vi "Main.vi"(11 "Error In":errorcluster) -> (15 "Error Out":errorcluster)   [LabVIEW 2022 SP3]
doc: "This VI has subpanel for sender and receiver. User can select the data type and transmission type for which communication has to take place from sender to receiver."
uses:
  Controls/Operation.ctl
  Controls/State Cluster.ctl
  Controls/Main Data Cluster.ctl
  Classes/Sender/Sender UI.vi
  Classes/Sender/Sender.lvclass
  Classes/Receiver/Receiver UI.vi
  Classes/Receiver/Receiver.lvclass
  Controls/User Event Operation.ctl
  Downloads/Sample PC Template/Sample PC Template/Typedefs/Data.ctl
  Downloads/Sample PC Template/Sample PC Template/Sample PC Template.lvlib
panel:
  in  "Help Button":bool
  # "Sender to Receiver Data Communication Model"
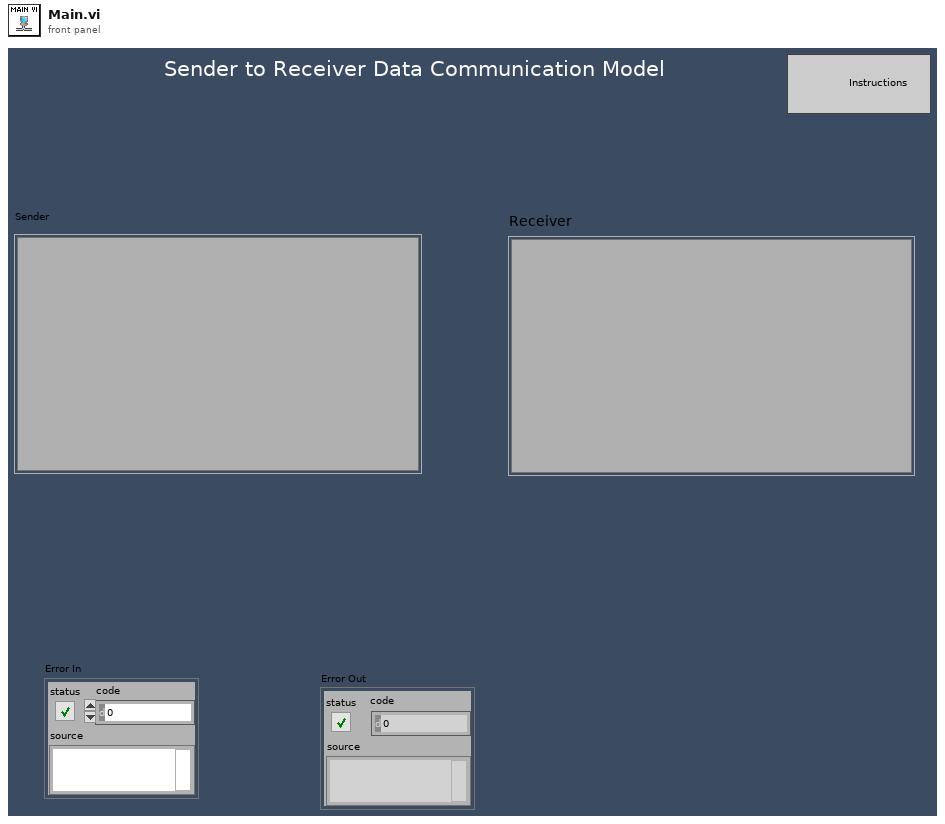
[diagram p1: front panel]
types:
  T1 = typedef "State Cluster.ctl" = cluster{"State":string, "Data":variant}
  T2 = typedef "Operation.ctl" = enum16{"Create", "Enqueue", "Enqueue N", "Enstack", "Dequeue", "Flush", "Release"}
  T3 = typedef "Sample PC Template.lvlib/Data.ctl" = cluster{"State":string, "Data":variant}
  T4 = typedef "User Event Operation.ctl" = enum16{"Obtain", "Generate", "Release"}
  T5 = typedef "Main Data Cluster.ctl" = cluster{"user event out":refnum<user-event>, "Sender Refnum":refnum<vi>, "Receiver refnum":refnum<vi>}
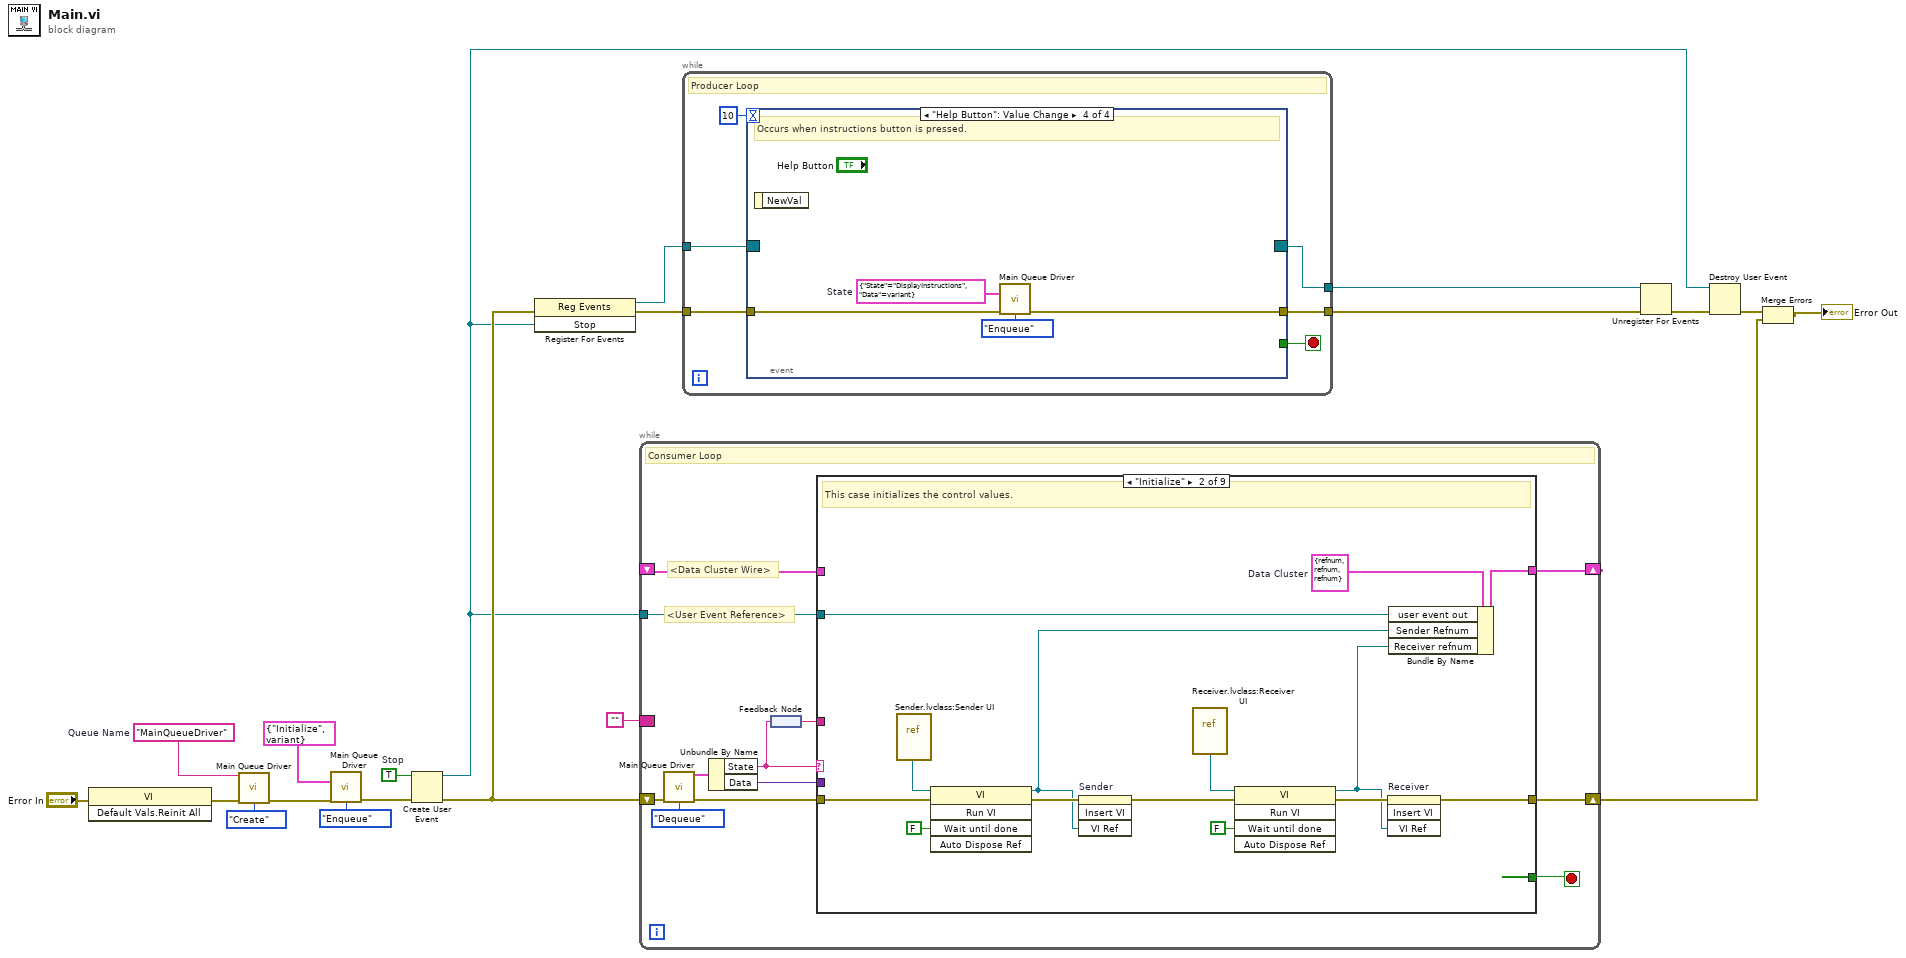
[diagram p0: block diagram]
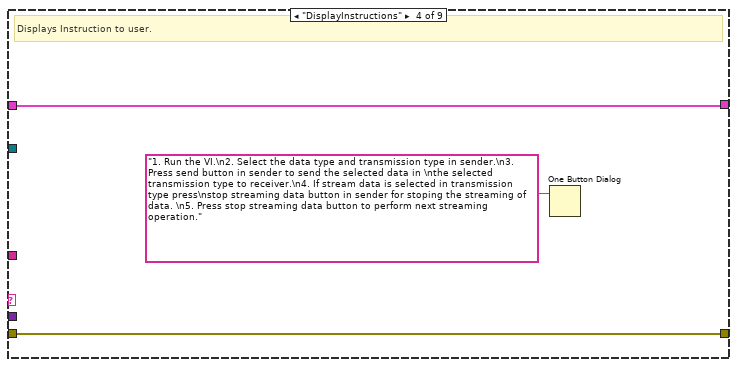
[diagram p4: hidden frame]
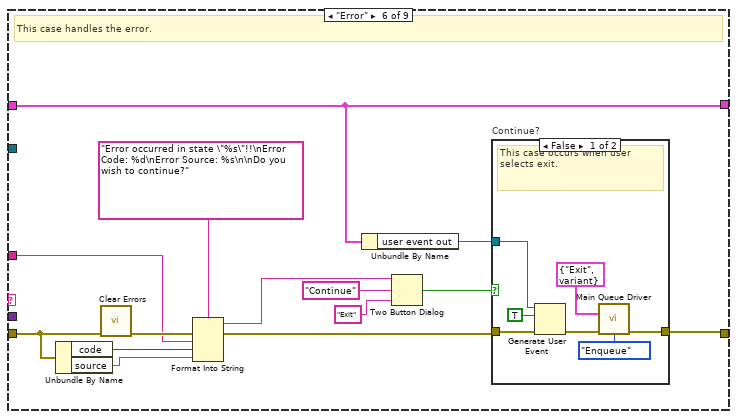
[diagram p6: hidden frame]
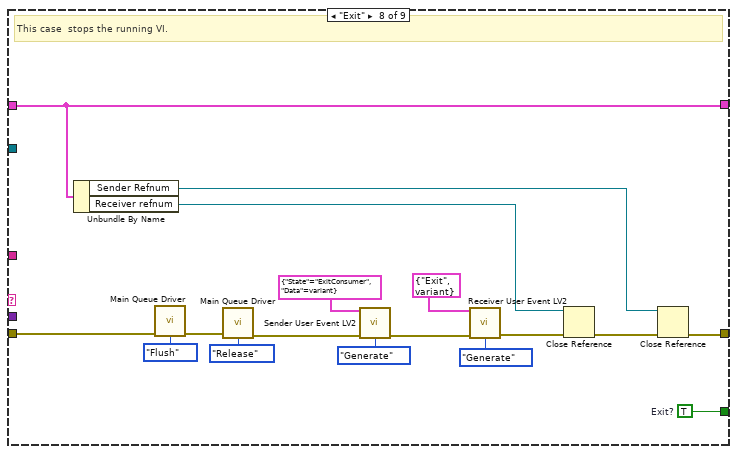
[diagram p9: hidden frame]
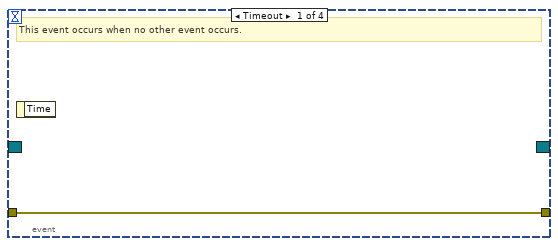
[diagram p11: hidden frame]
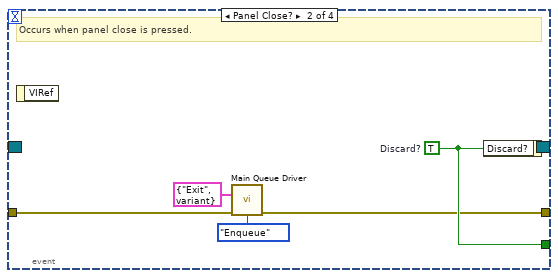
[diagram p12: hidden frame]
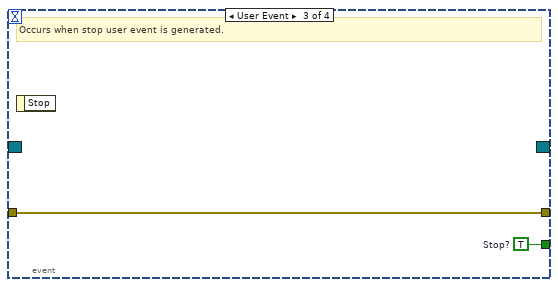
[diagram p13: hidden frame]
diagram:
  w14 = TRUE  # Stop
  w19 = "MainQueueDriver"  # Queue Name
  n1 = invoke class="VI" method="Default Vals.Reinit All"(error in="Error In") -> (error out=w1:errorcluster)  [unwired: 2 in, 2 out]
  n2 = call "Main Queue Driver.vi"("Queue Name"=w19, "Error In"=w1, "Operations"=Operation."Create") -> ("Error Out"=w18:errorcluster)  [unwired: 11 in, 1 out]
  n3 = call "Main Queue Driver.vi"("State"=T1 {"State"="Initialize", "Data"=variant}, "Error In"=w18, "Operations"=Operation."Enqueue") -> ("Error Out"=w15:errorcluster)  [unwired: 11 in, 1 out]
  n4 = Create User Event(user event datatype=w14, error in=w15) -> (user event=w3:refnum<user-event>, error out=w13:errorcluster)
  n5 = register-events(error in=w13, w3) -> (reference out=w11:refnum<event-registration>, error out=w12:errorcluster)  [unwired: 1 in]
  n6 = while {
    shift-right: [w26] -> w5
    shift-left: w13 -> [w31]
    border: "" -> [_]
    tunnel: w3 -> [w23]
    shift-right: [w22] -> _
    shift-left: _ -> [w24]
    stop <- w25 stop-if-true
    # "<Data Cluster Wire>"
    # "<User Event Reference>"
    # "Consumer Loop"
    n7 = call "Main Queue Driver.vi"("Error In"=w31, "Operations"=Operation."Dequeue") -> ("Dequeued Element"=w29:T1, "Error Out"=w30:errorcluster)  [unwired: 12 in]
    n8 = Unbundle By Name(w29) -> ("State"=w27:string, "Data"=w28:variant)
    n9 = feedback-in #1(w27) -> ()
    n10 = feedback #1() -> (w21:string)
    n11 = case shown="\"Initialize\"" w27 {
      tunnel: w30 -> [w34 w46 w50 w53 w55 w62 w79 w95 w98]
      tunnel: w28 -> [_ _ _ _ _ _ _ _ _]
      tunnel: [w34 w38 w50 w53 w55 w59 w79 w83 w98] -> w26
      tunnel: [_ _ _ _ _ _ _ w92 _] -> w25
      tunnel: w24 -> [w33 _ w49 w52 w54 w58 w78 w84 w97]
      tunnel: w23 -> [_ w48 _ _ _ _ _ _ _]
      tunnel: [w33 w47 w49 w52 w54 w58 w78 w84 w97] -> w22
      tunnel: w21 -> [_ _ _ _ _ w56 _ _ _]
      frame "/******** Initialization *********/" {
      }
      frame "Initialize" {
        w35 = T5 {"user event out"=refnum, "Sender Refnum"=refnum, "Receiver refnum"=refnum}  # Data Cluster
        # "This case initializes the control values."
        n12 = vi-ref "Sender.lvclass:Sender UI.vi"() -> (w45:refnum<vi>)
        n13 = invoke class="VI" method="Run VI"(reference=w45, error in=w46, "Wait until done"=FALSE ("Wait Until Done")) -> (reference out=w37:refnum<vi>, error out=w41:errorcluster)  [unwired: 2 in, 3 out]
        n14 = invoke on="Sender" class="SubPnl" method="Insert VI"(error in=w41, "VI Ref"=w37) -> (error out=w40:errorcluster)  [unwired: 2 in, 3 out]
        n15 = vi-ref "Receiver.lvclass:Receiver UI.vi"() -> (w44:refnum<vi>)
        n16 = invoke class="VI" method="Run VI"(reference=w44, error in=w40, "Wait until done"=FALSE ("Wait Until Done")) -> (reference out=w36:refnum<vi>, error out=w39:errorcluster)  [unwired: 2 in, 3 out]
        n17 = invoke on="Receiver" class="SubPnl" method="Insert VI"(error in=w39, "VI Ref"=w36) -> (error out=w38:errorcluster)  [unwired: 2 in, 3 out]
        n18 = Bundle By Name(cluster=w35, "user event out"=w48, "Sender Refnum"=w37, "Receiver refnum"=w36) -> (w47:T5)
      }
      frame "/****** Display Instruction ******/" {
      }
      frame "DisplayInstructions" {
        # "Displays Instruction to user."
        n19 = One Button Dialog(message="1. Run the VI.\n2. Select the data type and transmission type in sender.\n3. Press send button in sender to send the selected data in \nthe selected transmission type to receiver.\n4. If stream data is selected in transmission type press\nstop streaming data button in sender for stoping the streaming of data. \n5. Press stop streaming data button to perform next streaming operation.") -> ()  [unwired: 1 in, 1 out]
      }
      frame "/******* Error Handling *******/" {
      }
      frame "Error" {
        # "This case handles the error."
        n20 = Unbundle By Name(w62) -> ("code"=w61:i32, "source"=w60:string)
        n21 = call <vilib>:"Clear Errors.vi"("error in (no error)"=w62) -> ("error out"=w69:errorcluster)  [unwired: 5 in, 1 out]
        n22 = Format Into String(format string="Error occurred in state \"%s\"!!\nError Code: %d\nError Source: %s\n\nDo you wish to continue?", error in=w69, w56, w61, w60) -> (resulting string=w67:string, error out=w64:errorcluster)  [unwired: 1 in]
        n23 = Unbundle By Name(w58) -> ("user event out"=w57:refnum<user-event>)
        n24 = Two Button Dialog(message=w67, 1:"Exit" ("F button name (\"Cancel\")"), 2:"Continue" ("T button name (\"OK\")")) -> (T button?=w63:bool)
        n25 = case "Continue?" shown="False" w63 {
          tunnel: w64 -> [w76 w77]
          tunnel: [w72 w77] -> w59
          tunnel: w57 -> [w74 _]
          frame False {
            # "This case occurs when user selects exit."
            n26 = Generate User Event(user event=w74, event data cluster=TRUE ("event data"), error in=w76) -> (error out=w73:errorcluster)  [unwired: 1 in, 1 out]
            n27 = call "Main Queue Driver.vi"("State"=T1 {"State"="Exit", "Data"=variant}, "Error In"=w73, "Operations"=Operation."Enqueue") -> ("Error Out"=w72:errorcluster)  [unwired: 11 in, 1 out]
          }
          frame True {
            # "This case occurs when user selects to continue."
          }
        }
      }
      frame "/******* Exit ********/" {
      }
      frame "Exit" {
        w92 = TRUE  # Exit?
        # "This case  stops the running VI."
        n28 = Unbundle By Name(w84) -> ("Sender Refnum"=w80:refnum<vi>, "Receiver refnum"=w81:refnum<vi>)
        n29 = call "Main Queue Driver.vi"("Error In"=w95, "Operations"=Operation."Flush") -> ("Error Out"=w93:errorcluster)  [unwired: 12 in, 1 out]
        n30 = call "Main Queue Driver.vi"("Error In"=w93, "Operations"=Operation."Release") -> ("Error Out"=w91:errorcluster)  [unwired: 12 in, 1 out]
        n31 = call "Sender User Event LV2.vi"("Data"=T3 {"State"="ExitConsumer", "Data"=variant}, "Error In"=w91, "Operation"=User_Event_Operation."Generate") -> ("Error Out"=w90:errorcluster)  [unwired: 11 in, 1 out]
        n32 = call "Receiver User Event LV2.vi"("Data"=T3 {"State"="Exit", "Data"=variant}, "Error In"=w90, "Operation"=User_Event_Operation."Generate") -> ("Error Out"=w89:errorcluster)  [unwired: 11 in, 1 out]
        n33 = Close Reference(reference=w81, error in (no error)=w89) -> (error out=w82:errorcluster)
        n34 = Close Reference(reference=w80, error in (no error)=w82) -> (error out=w83:errorcluster)
      }
      frame Default {
        # "Occurs if any developer error."
      }
    }
  }
  n35 = while {
    tunnel: w12 -> [w103]
    tunnel: w11 -> [w102]
    tunnel: [w101] -> w9
    tunnel: [w100] -> w8
    stop <- w99 stop-if-true
    # "Producer Loop"
    n36 = event shown="[3] \"Help Button\": Value Change" {
      selector: w102 -> [_ _ _ _]
      dyn-events: [_ _ _ _] -> w101
      timeout: 10 -> [_ _ _ _]
      tunnel: w103 -> [w105 w109 w112 w116]
      tunnel: [w105 w108 w112 w115] -> w100
      tunnel: [_ w110 w111 _] -> w99
      event Timeout {
        # "This event occurs when no other event occurs."
        n37 = event-data() -> ()  [unwired: 1 in, 1 out]
      }
      event Panel Close? {
        w110 = TRUE  # Discard?
        # "Occurs when panel close is pressed."
        n38 = event-data() -> ()  [unwired: 1 in, 1 out]
        n39 = call "Main Queue Driver.vi"("State"=T1 {"State"="Exit", "Data"=variant}, "Error In"=w109, "Operations"=Operation."Enqueue") -> ("Error Out"=w108:errorcluster)  [unwired: 11 in, 1 out]
        n40 = event-data("Discard?"=w110) -> ()  [unwired: 1 in, 1 out]
      }
      event User Event {
        w111 = TRUE  # Stop?
        # "Occurs when stop user event is generated."
        n41 = event-data() -> ()  [unwired: 1 in, 1 out]
      }
      event "Help Button": Value Change {
        w113 = T1 {"State"="DisplayInstructions", "Data"=variant}  # State
        # "Occurs when instructions button is pressed."
        n42 = event-data() -> ()  [unwired: 1 in, 1 out]
        n43 = call "Main Queue Driver.vi"("State"=w113, "Error In"=w116, "Operations"=Operation."Enqueue") -> ("Error Out"=w115:errorcluster)  [unwired: 11 in, 1 out]
      }
    }
  }
  n44 = Unregister For Events(event registration refnum=w9, error in=w8) -> (error out=w7:errorcluster)
  n45 = Destroy User Event(user event=w3, error in=w7) -> (error out=w6:errorcluster)
  n46 = Merge Errors(w6, w5) -> (→"Error Out":errorcluster)
